vi "Invalid_Commands_Window.vi"(1 "Invalid Commands":string[](array[string])) -> ()   [LabVIEW 2011]
panel:
  in  "OK":bool
  in  "Invalid Commands List":i32(listbox)
  # "The following invalid commands were found in the growth sequence:"
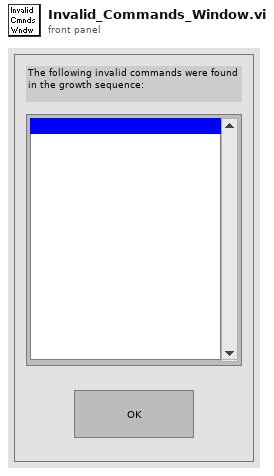
[diagram p1: front panel]
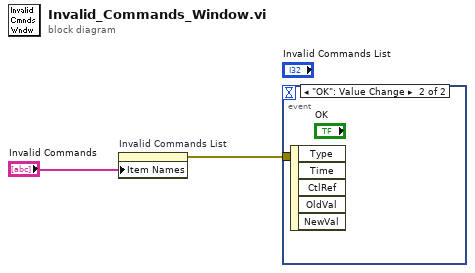
[diagram p0: block diagram]
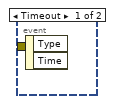
[diagram p2: hidden frame]
diagram:
  n1 = property on="Invalid Commands List" class="LstBox (strict)"("Item Names"="Invalid Commands") -> (error out=w1:errorcluster)  [unwired: 2 in, 1 out]
  n2 = event shown="[1] \"OK\": Value Change" {
    selector: _ -> [_ _]
    dyn-events: _ -> [_ _]
    timeout: _ -> [_ _]
    tunnel: w1 -> [_ _]
    event Timeout {
      n3 = event-data() -> ()  [unwired: 1 in, 2 out]
    }
    event "OK": Value Change {
      n4 = event-data() -> ()  [unwired: 1 in, 5 out]
    }
  }
